vi "ClassAttributes_AddClassAttributes.vi"(7 "Action":T3=enum."GeneratePattern", 8 "error in (no error)":errorcluster, 10 "DataIn":variant, 11 "ClassRefToActOn":refnum<vi>) -> (0 "error out":errorcluster, 1 "Name":string, 2 "DataOut":variant, 3 "Cancelled":bool)   [LabVIEW 2012]
uses:
  <resource>/Framework/Providers/Open_GDS/ClassProviders/Provider_BaseClassInterface/BaseProvider_SubVIs/BaseProvider_DesignPatternsActions.ctl
  <resource>/Framework/Providers/Open_GDS/ClassProviders/Common/CommonVIs/CommonVIs_AttributeDataType.ctl
  <resource>/Framework/Providers/Open_GDS/ClassProviders/Common/LvClass_class/GDSLvClass_ProviderTypes.ctl
  <resource>/Framework/Providers/Open_GDS/ClassProviders/Common/ScriptingFunctions/Scripting_ConnectorPanePatternType.ctl
  <vilib>/picture/picture.llb/imagedata.ctl
  <resource>/Framework/Providers/Open_GDS/ClassProviders/Provider_LvNativeClass/ClassWriterNative_class/ClassWriterNative.lvclass
  <resource>/Framework/Providers/Open_GDS/ClassProviders/Provider_BaseClassInterface/CreateMethodData.ctl
  <resource>/Framework/Providers/Open_GDS/ClassProviders/Provider_EndevoGOOP300/GOOP300_SubVIs/GOOP300_MethodScopeType.ctl
  <resource>/Framework/Providers/Open_GDS/ClassProviders/Provider_LvNativeClass/ClassWriterNative_class/IconDetails.ctl
  <resource>/Framework/Providers/Open_GDS/ClassProviders/Provider_LvNativeClass/ClassWriterNative_class/IconSize.ctl
  <resource>/Framework/Providers/Open_GDS/ClassProviders/Provider_BaseClassInterface/ClassWriter_class/ClassWriter.lvclass
panel:
  in  "_Cancel":bool
  in  "_OK":bool
  in  "ProcessName":T2(array[cluster]) caption="Attributes to add (can be empty)\nName                                              Array?      Data Type" {"Array?" items=["No", "1D", "2D", "3D"]}
  # "Class Attributes"
  # "Create"
  # "Get"
  # "Set"
  # "method"
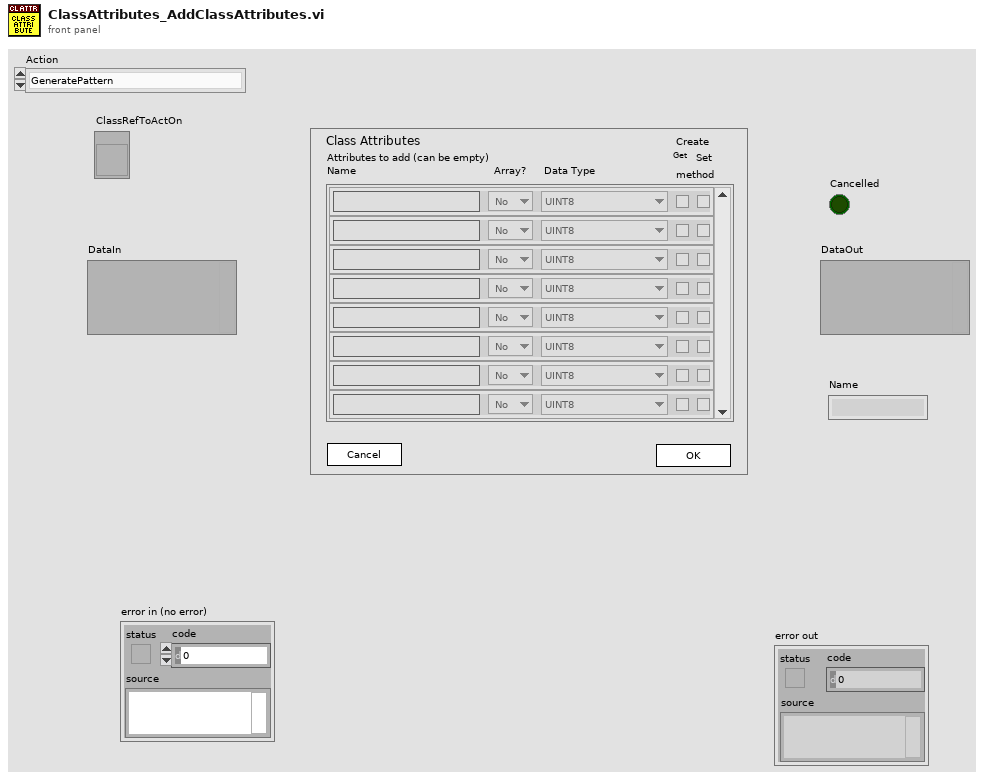
[diagram p1: front panel]
types:
  T1 = typedef "CommonVIs_AttributeDataType.ctl" = enum16{"UINT8", "INT8", "UINT16", "INT16", "UINT32", "INT32", "UINT64", "INT64", "SGL", "DBL", "EXT", "CSG", "CDB", "CXT", "TimeStamp", "STRING", "PATH", "BOOL", "ENUM", "RefNum", "VIRefNum", "ClassRefNum", "Cluster", "Variant", "TypeRef", "Waveform", "LabVIEW Object", "Other"}
  T2 = cluster{"Name":string, "Array?":u16, "AttributeDataType":T1, "GetMethod":bool, "SetMethod":bool}[]
  T3 = typedef "BaseProvider_DesignPatternsActions.ctl" = enum16{"AddPatternDialog", "GeneratePattern", "RemovePattern", "CreatePatternMethod", "UpdatePattern"}
  T4 = typedef "GDSLvClass_ProviderTypes.ctl" = enum16{"UnKnown(LabVOOP)", "Native", "EndevoGOOP3", "OpenG(RootObject)", "OpenG(OpenG_Object)", "EndevoGOOP4", "JKI1"}
  T5 = cluster{"Application":refnum<vi>, "SupportFolder":path, "TemplateName":string, "ClassProvider":T4, "ProtectedFolder":path, "UtilsFolder":path, "ProtectedFolderRef":refnum<vi>, "UtilsFolderRef":refnum<vi>, "ClassName":string, "GetClassAttributes.vi":path, "ClassAttributes.ctl":path, "GetClassAttributesRef":refnum<vi>, "ClassAttributesRef":refnum<vi>, "ProcessIdRef":refnum<vi>, "Data":cluster{"Name":string, "Array?":u16, "AttributeDataType":T1, "GetMethod":bool, "SetMethod":bool}[], "Singleton":bool, "VI_ToFind":path, "MethodTemplate":path, "VI":refnum<vi>, "GetObjectStatus":path}
  T6 = cluster{"ProcessName":cluster{"Name":string, "Array?":u16, "AttributeDataType":T1, "GetMethod":bool, "SetMethod":bool}[]}
  T7 = cluster{"Cancelled":bool, "Files":path[], "ClassPath":path, "DataOut":variant}
  T8 = enum32{"invalid lock state", "Not Locked", "Locked (No Password)", "Password-protected"}
  T9 = typedef "imagedata.ctl" = cluster{"image type":i32, "image depth":i32, "image":u8[], "mask":u8[], "colors":u32[], "Rectangle":cluster{"left":i16, "top":i16, "right":i16, "bottom":i16}}
  T10 = typedef "ClassWriter.lvclass/CreateMethodData.ctl" = cluster{"MethodName":string, "RelativeMethodPath":path, "MethodDescription":string, "Scope/Visibility":T11, "MethodTemplateName":string, "IconOut":u8[][], "RelativeProjectClassPath":string, "OpenViAfterCreation":bool, "DynamicDispatchVi":bool, "ExtraCreateParameters":variant, "MustOverride":bool, "MustCallParent":bool, "IconDetails":T12, "AF-Option":variant, "TemplatePath":path}
  T11 = typedef "GOOP300_MethodScopeType.ctl" = enum16{"Use Parent Folder Scope", "Public", "Protected", "Private", "Community"}
  T12 = typedef "ClassWriterNative.lvclass/IconDetails.ctl" = cluster{"IconSize":T13, "ImageRows(32)":i32, "ConnectorPaneHeight":i32[]}
  T13 = typedef "ClassWriterNative.lvclass/IconSize.ctl" = enum16{"Full", "1 c-term high", "2 c-term high", "3 c-term high"}
  T14 = typedef "GDSLvCLass_ClassSettingsType.ctl" = cluster{"ClassProviderName":string, "ClassTemplateUsed":string, "ClassTemplateVersion":string, "ClassDescription":string, "PlugIns":T15[], "ConnectorPanePattern":string}
  T15 = typedef "GDSLvClass_PlugIn.ctl" = cluster{"Type":T16, "ID":string, "Version":string, "Path":path, "Name":string, "Data":variant}
  T16 = typedef "GDSLvClass_PlugInTypes.ctl" = enum16{"DesignPattern", "MethodTypes"}
  T17 = enum32{"invalid scope", "public", "private", "protected"}[]
  T18 = typedef "Scripting_ConnectorPanePatternType.ctl" = u16
  T19 = typedef "GDSLvClass_IconSettingsType.ctl" = cluster{"Frame":u32, "Frame thickness":u8, "Header Background":u32, "Header Text":u32, "ColorPublic":u32, "ColorProtected":u32, "ColorPrivate":u32, "Body Text":u32, "ClassBodyIcon":string}
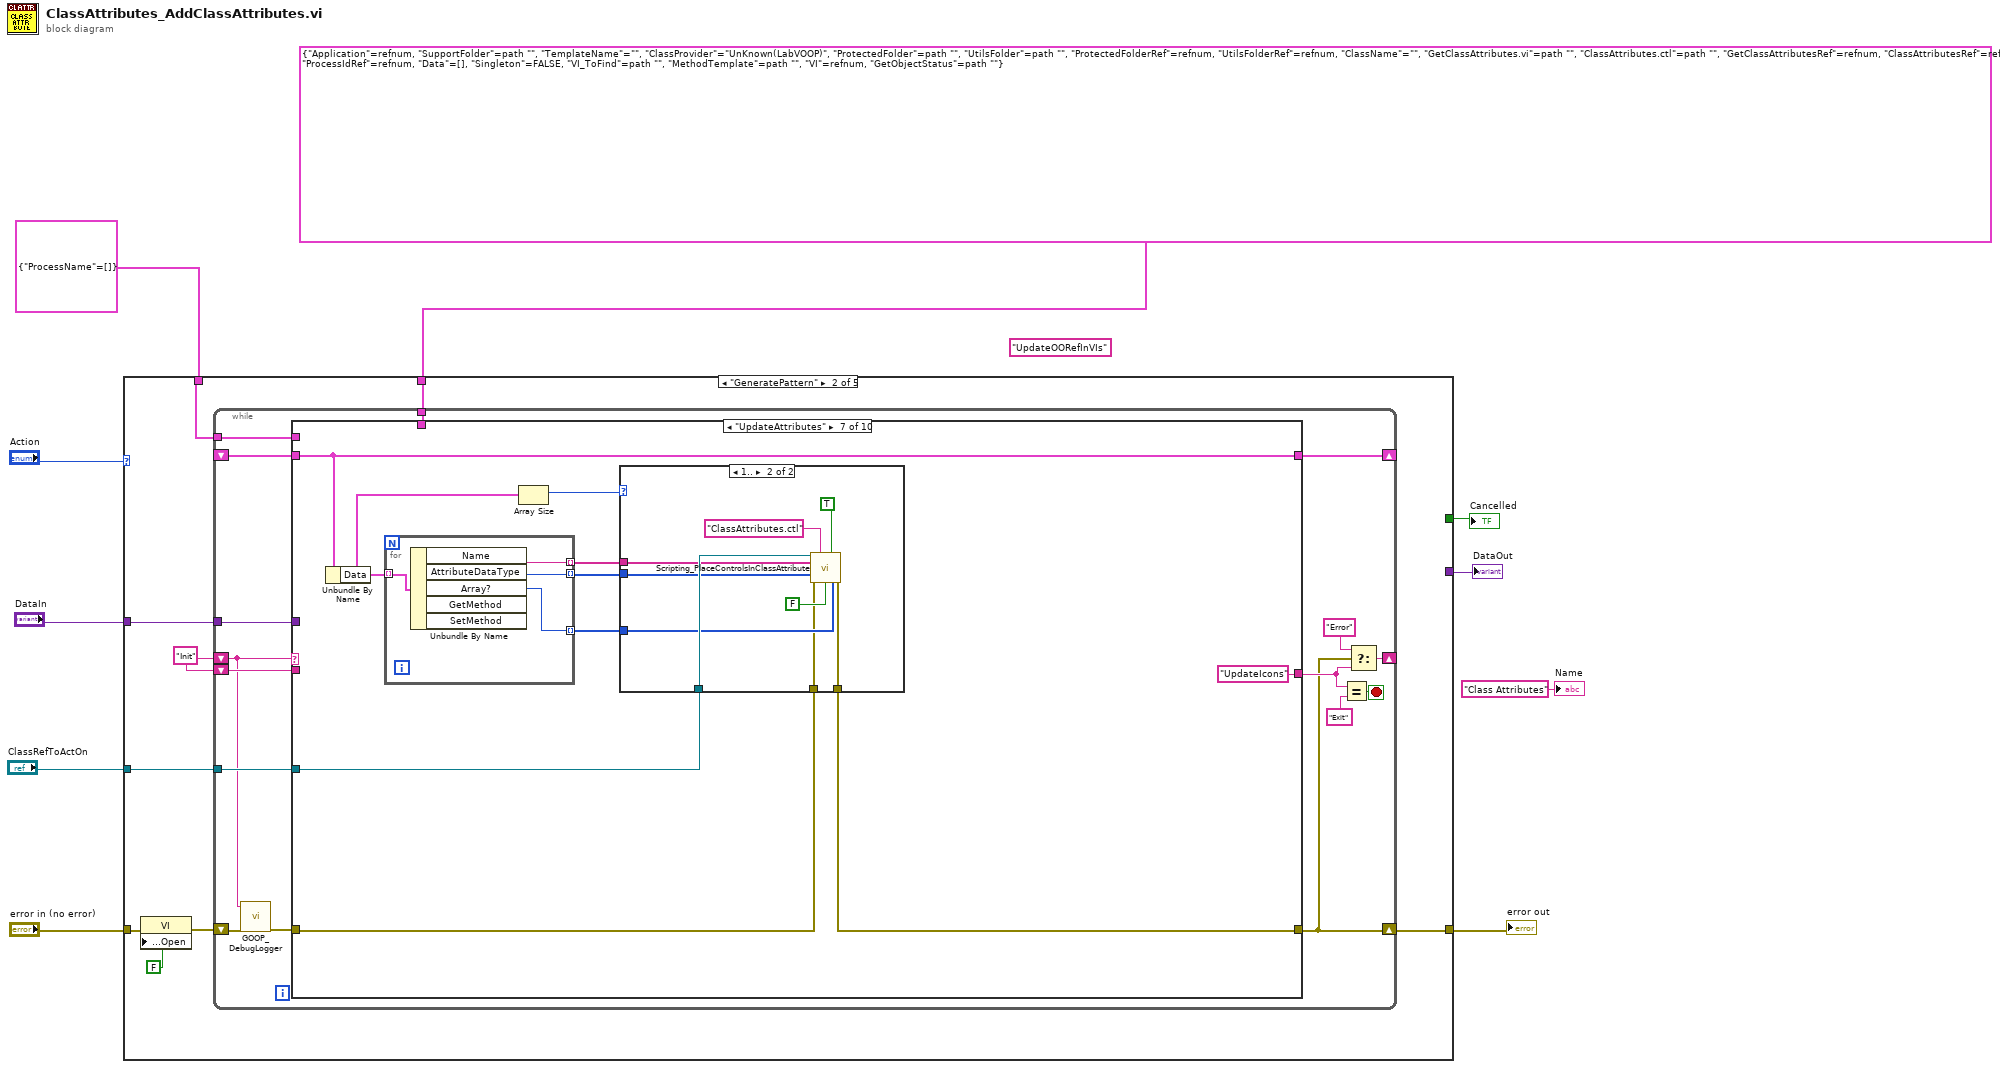
[diagram p0: block diagram]
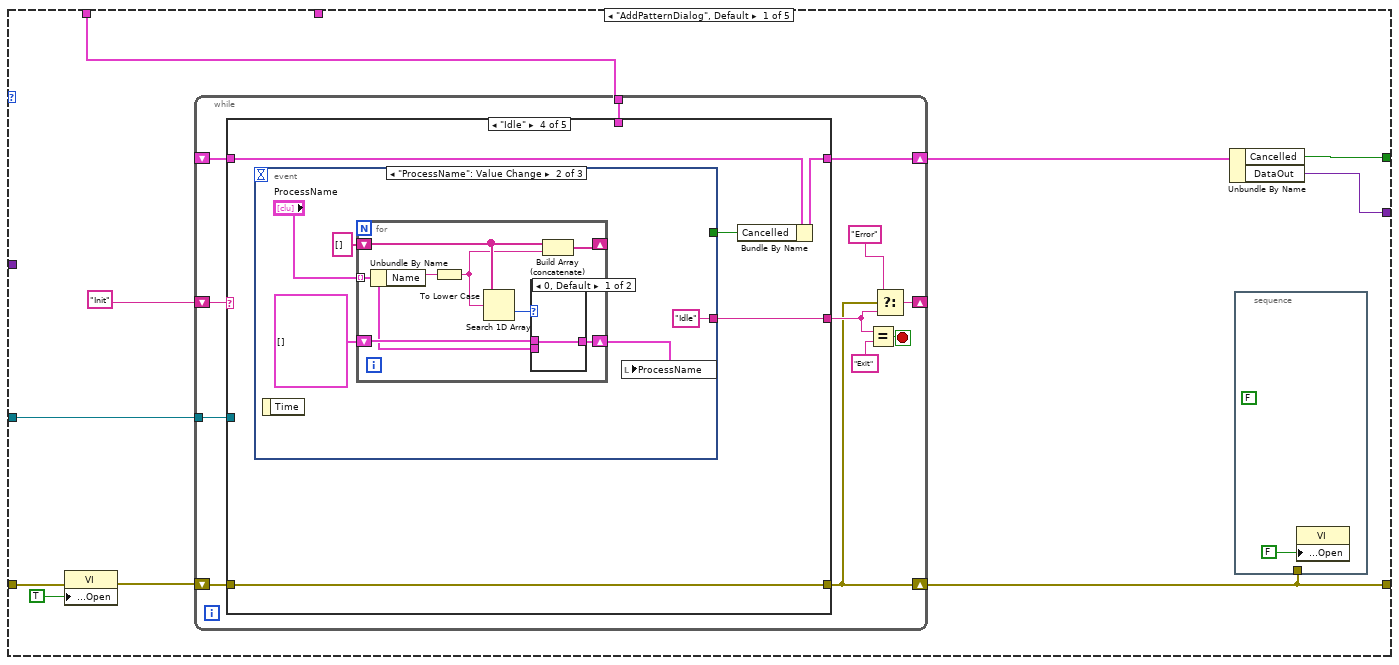
[diagram p2: hidden frame]
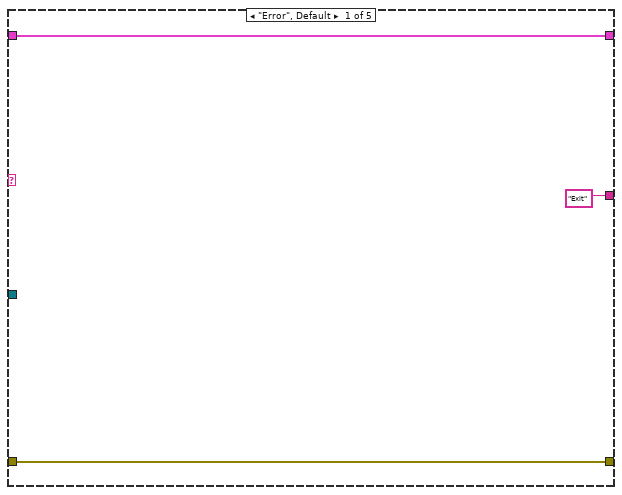
[diagram p3: hidden frame]
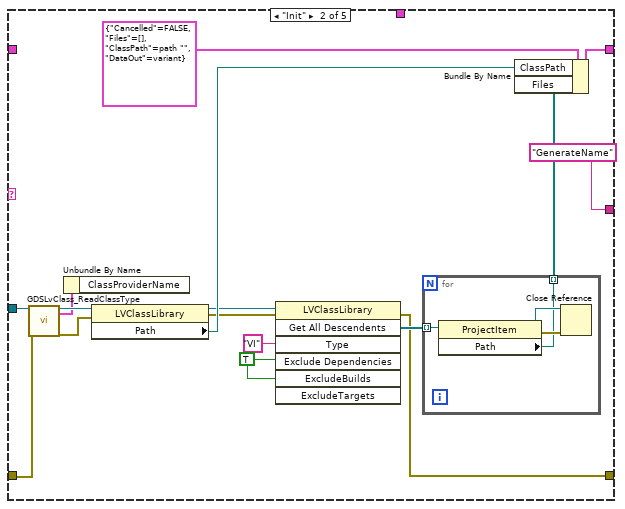
[diagram p4: hidden frame]
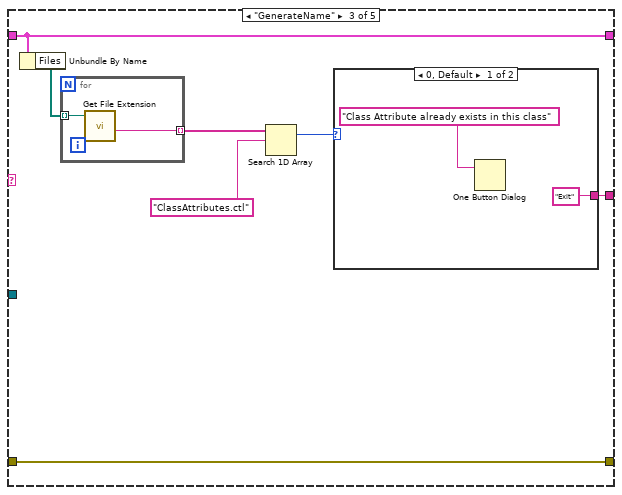
[diagram p5: hidden frame]
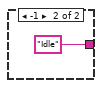
[diagram p6: hidden frame]
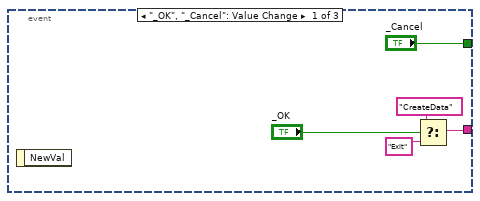
[diagram p7: hidden frame]
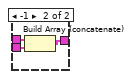
[diagram p8: hidden frame]
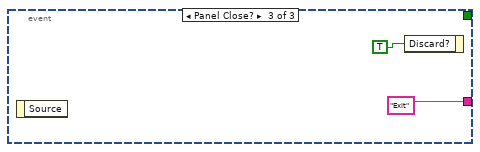
[diagram p9: hidden frame]
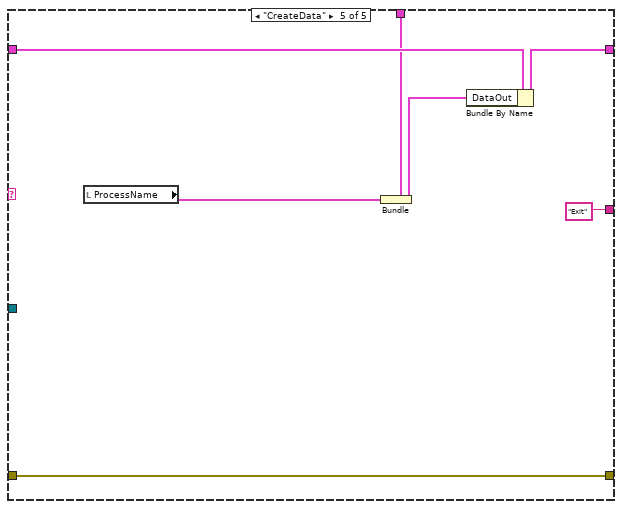
[diagram p10: hidden frame]
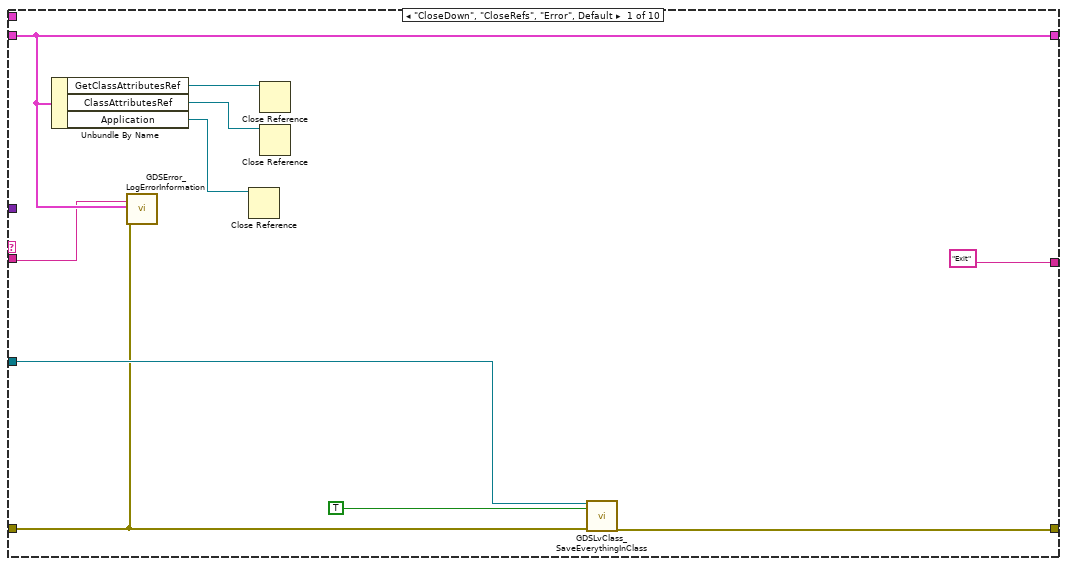
[diagram p11: hidden frame]
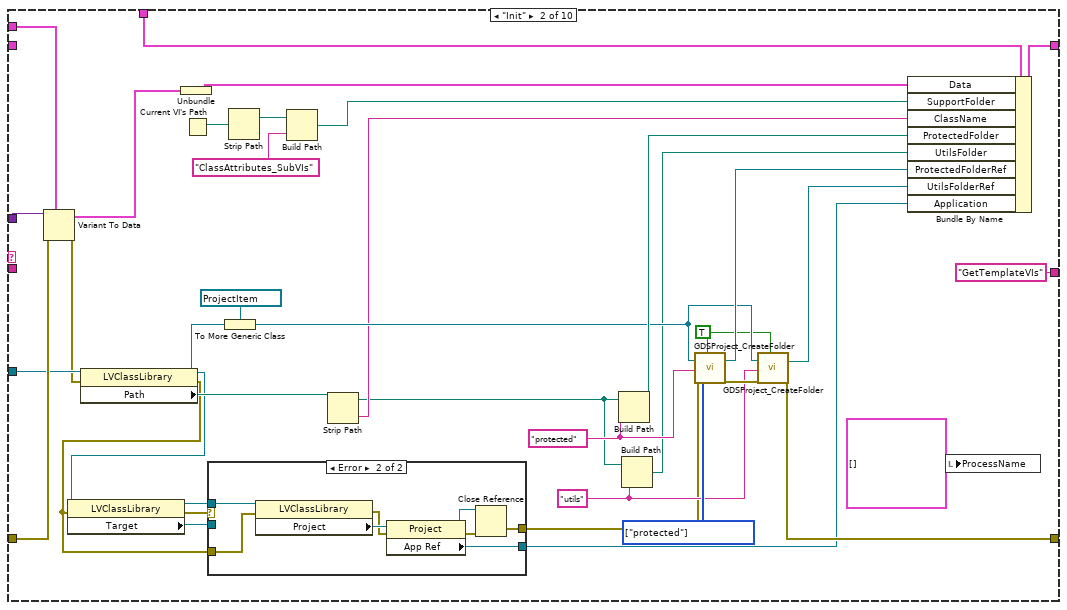
[diagram p12: hidden frame]
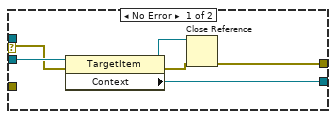
[diagram p13: hidden frame]
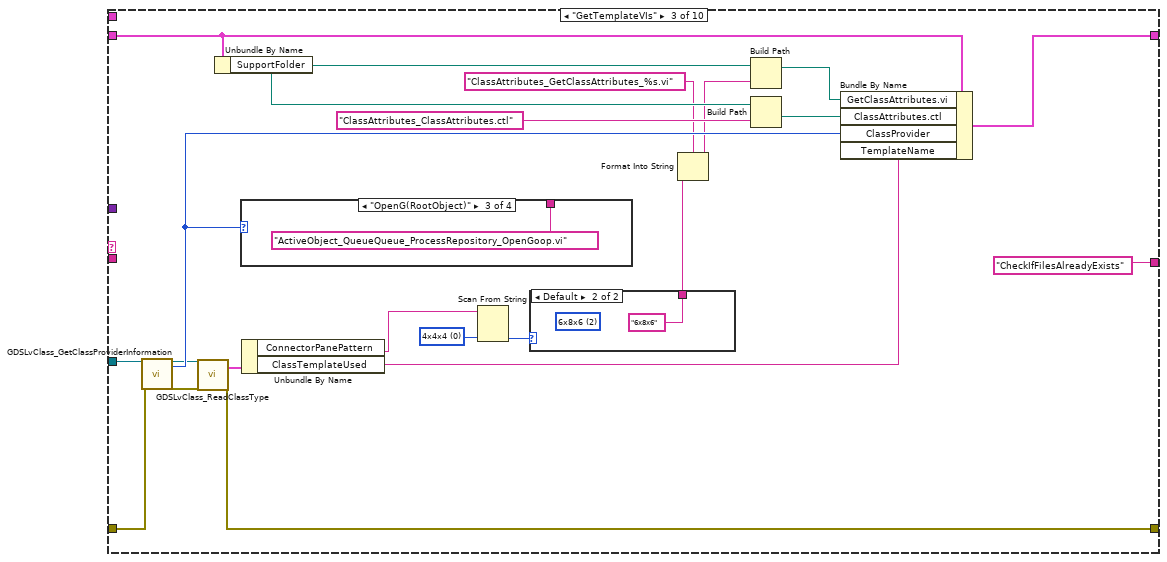
[diagram p14: hidden frame]
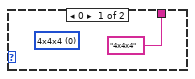
[diagram p15: hidden frame]
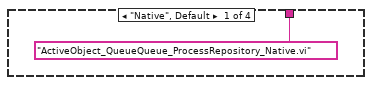
[diagram p16: hidden frame]
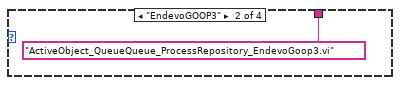
[diagram p17: hidden frame]
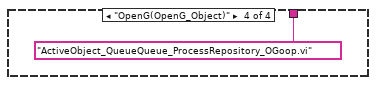
[diagram p18: hidden frame]
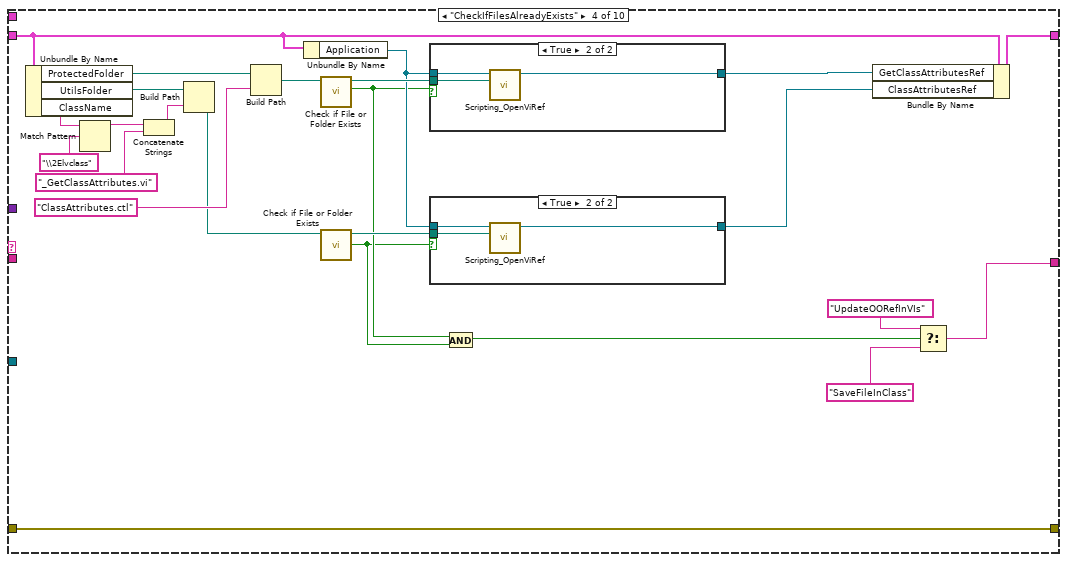
[diagram p19: hidden frame]
diagram:
  (unwired) "UpdateOORefInVIs"
  n1 = case shown="\"GeneratePattern\"" "Action" {
    tunnel: "error in (no error)" -> [w19 w107 w531 w622 w623]
    tunnel: [w16 w113 w537 w622 w623] -> w8
    tunnel: "ClassRefToActOn" -> [w14 w109 w533 _ _]
    tunnel: [w13 _ _ _ _] -> w6
    tunnel: [w12 _ _ _ _] -> w5
    tunnel: T6 {"ProcessName"=[]} ("output cluster") -> [w11 w111 w535 _ _]
    tunnel: "DataIn" -> [_ w112 w536 _ _]
    tunnel: T5 {"Application"=refnum, "SupportFolder"=path "", "TemplateName"="", "ClassProvider"=enum."UnKnown(LabVOOP)", "ProtectedFolder"=path "", "UtilsFolder"=path "", "ProtectedFolderRef"=refnum, "UtilsFolderRef"=refnum, "ClassName"="", "GetClassAttributes.vi"=path "", "ClassAttributes.ctl"=path "", "GetClassAttributesRef"=refnum, "ClassAttributesRef"=refnum, "ProcessIdRef"=refnum, "Data"=[], "Singleton"=FALSE, "VI_ToFind"=path "", "MethodTemplate"=path "", "VI"=refnum, "GetObjectStatus"=path ""} -> [_ w110 w534 _ _]
    frame "AddPatternDialog", Default {
      n2 = property class="VI"(error in=w19, "Front Panel.Open"=TRUE ("Front Panel Window:Open")) -> (error out=w18:errorcluster)  [unwired: 1 in, 1 out]
      n3 = while {
        shift-right: [w26] -> w16
        shift-left: w18 -> [w33]
        shift-right: [w31] -> _
        shift-left: "Init" -> [w32]
        shift-right: [w25] -> w15
        shift-left: _ -> [w24]
        tunnel: w14 -> [w23]
        tunnel: w11 -> [w22]
        stop <- w30 stop-if-true
        n4 = case shown="\"Idle\"" w32 {
          tunnel: w33 -> [w36 w39 w60 w72 w100]
          tunnel: [w36 w48 w60 w72 w100] -> w26
          tunnel: ["Exit" "GenerateName" w62 w73 "Exit"] -> w27
          tunnel: [w34 w46 w61 w71 w102] -> w25
          tunnel: w24 -> [w34 _ w61 w69 w104]
          tunnel: w23 -> [_ w41 _ _ _]
          tunnel: w22 -> [_ _ _ _ w99]
          frame "Error", Default {
          }
          frame "Init" {
            w50 = TRUE ("ExcludeDependencies")
            n5 = call <resource>:"GDSLvClass_ReadClassType.vi"("Class Refnum In"=w41, "error in (no error)"=w39) -> ("Class Refnum Out"=w40:refnum<vi>, "ClassSettings"=w37:T14, "error out"=w38:errorcluster)  [unwired: 15 in]
            n6 = Unbundle By Name(w37) -> ()  [unwired: 1 out]
            n7 = property class="LVClassLibrary"(reference=w40, error in=w38) -> (reference out=w43:refnum<vi>, error out=w42:errorcluster, "Path"=w45:path)
            n8 = invoke class="LVClassLibrary" method="Get All Descendents"(reference=w43, error in=w42, "Type"="VI", "Exclude Dependencies"=w50, "ExcludeBuilds"=w50) -> (error out=w48:errorcluster, "All Descendents"=w49:refnum<vi>[])  [unwired: 2 in, 5 out]
            n9 = for {
              tunnel: w49 -> [w56] mode=indexing
              tunnel: [w53] -> w44 mode=indexing
              n10 = property class="ProjectItem"(reference=w56) -> (reference out=w54:refnum<vi>, error out=w55:errorcluster, "Path"=w53:path)  [unwired: 1 in]
              n11 = Close Reference(reference=w54, error in (no error)=w55) -> ()  [unwired: 1 out]
            }
            n12 = Bundle By Name(cluster=T7 {"Cancelled"=FALSE, "Files"=[], "ClassPath"=path "", "DataOut"=variant}, "ClassPath"=w45, "Files"=w44) -> (w46:T7)
          }
          frame "GenerateName" {
            n13 = Unbundle By Name(w61) -> ("Files"=w63:path[])
            n14 = for {
              tunnel: w63 -> [w68] mode=indexing
              tunnel: [w67] -> w59 mode=indexing
              n15 = call <vilib>:"Get File Extension.vi"("file"=w68) -> ("filename without extension"=w67:string)  [unwired: 7 in, 3 out]
            }
            n16 = Search 1D Array(1D array=w59, element="ClassAttributes.ctl") -> (index of element=w57:i32)  [unwired: 1 in]
            n17 = case shown="0, Default" w57 {
              tunnel: ["Exit" "Idle"] -> w62
              frame 0, Default {
                n18 = One Button Dialog(message="Class Attribute already exists in this class") -> ()  [unwired: 1 in, 1 out]
              }
              frame -1 {
              }
            }
          }
          frame "Idle" {
            n19 = event shown="[1] \"ProcessName\": Value Change" {
              selector: _ -> [_ _ _]
              dyn-events: _ -> [_ _ _]
              timeout: _ -> [_ _ _]
              tunnel: [w77 "Idle" "Exit"] -> w73
              tunnel: ["_Cancel" _ _] -> w70
              event "_OK", "_Cancel": Value Change {
                n20 = event-data() -> ()  [unwired: 1 in, 1 out]
                n21 = Select(t="CreateData", s="_OK", f="Exit") -> (s? t:f=w77:string)
              }
              event "ProcessName": Value Change {
                n22 = event-data() -> ()  [unwired: 1 in, 1 out]
                n23 = for {
                  tunnel: "ProcessName" -> [w85] mode=indexing
                  shift-right: [w91] -> _
                  shift-left: string[] [] -> [w89]
                  shift-right: [w84] -> w79
                  shift-left: T2 [] -> [w86]
                  n24 = Unbundle By Name(w85) -> ("Name"=w90:string)
                  n25 = To Lower Case(string=w90) -> (all lower case string=w88:string)
                  n26 = Search 1D Array(1D array=w89, element=w88) -> (index of element=w87:i32)  [unwired: 1 in]
                  n27 = case shown="0, Default" w87 {
                    tunnel: w86 -> [w92 w95]
                    tunnel: w85 -> [_ w94]
                    tunnel: [w92 w93] -> w84
                    frame 0, Default {
                    }
                    frame -1 {
                      n28 = Build Array (concatenate)(w95, w94) -> (w93:T2)
                    }
                  }
                  n29 = Build Array (concatenate)(w89, w88) -> (w91:string[])
                }
                n30 = local write "ProcessName"(w79) -> ()
              }
              event Panel Close? {
                n31 = event-data() -> ()  [unwired: 1 in, 1 out]
                n32 = event-data("Discard?"=TRUE) -> ()  [unwired: 1 in, 1 out]
              }
            }
            n33 = Bundle By Name(cluster=w69, "Cancelled"=w70) -> (w71:T7)
          }
          frame "CreateData" {
            n34 = local read "ProcessName"() -> (w98:T2)
            n35 = Bundle(cluster=w99, "ProcessName"=w98) -> (w103:T6)
            n36 = Bundle By Name(cluster=w104, "DataOut"=w103) -> (w102:T7)
          }
        }
        n37 = Equal?(x=w27, y="Exit") -> (x = y?=w30:bool)
        n38 = Select(t="Error", s=w26, f=w27) -> (s? t:f=w31:string)
      }
      n39 = Unbundle By Name(w15) -> ("Cancelled"=w13:bool, "DataOut"=w12:variant)
      n40 = stacked-sequence {
        tunnel: w16 -> [_]
        frame #0 {
          (unwired) FALSE ("Visible")
          n41 = property class="VI"("Front Panel.Open"=FALSE ("Front Panel Window:Open")) -> ()  [unwired: 2 in, 2 out]
        }
      }
    }
    frame "GeneratePattern" {
      w105 = "Init"
      n42 = property class="VI"(error in=w107, "Front Panel.Open"=FALSE ("Front Panel Window:Open")) -> (error out=w106:errorcluster)  [unwired: 1 in, 1 out]
      n43 = while {
        shift-right: [w124] -> w113
        shift-left: w106 -> [w116]
        shift-right: [w129] -> _
        shift-left: w105 -> [w114]
        shift-right: [w123] -> _
        shift-left: _ -> [w122]
        tunnel: w112 -> [w121]
        tunnel: w111 -> [w120]
        tunnel: w110 -> [w119]
        tunnel: w109 -> [w118]
        shift-left: w105 -> [w117]
        stop <- w128 stop-if-true
        n44 = call <resource>:"GOOP_DebugLogger.vi"("error in (no error)"=w116, "State"=w114) -> ("error out"=w115:errorcluster)  [unwired: 9 in]
        n45 = case shown="\"UpdateAttributes\"" w114 {
          tunnel: w115 -> [w130 w171 w209 w232 w274 w303 w312 w336 w389 w476]
          tunnel: [w135 w156 w202 w232 w276 w297 w311 w335 w386 w461] -> w124
          tunnel: ["Exit" "GetTemplateVIs" "CheckIfFilesAlreadyExists" w218 "UpdateOORefInVIs" "UpdateAttributes" "UpdateIcons" "CreateMethods" w381 "CloseRefs"] -> w125
          tunnel: [w132 w175 w205 w228 w291 w304 w317 w338 w378 w460] -> w123
          tunnel: w122 -> [w132 _ w208 w229 w259 w304 w317 w338 w379 w460]
          tunnel: w121 -> [_ w174 _ _ _ _ _ _ _ _]
          tunnel: w120 -> [_ w173 _ _ _ _ _ _ _ _]
          tunnel: w119 -> [_ w172 _ _ _ _ _ _ _ _]
          tunnel: w118 -> [w134 w170 w210 _ _ w302 w316 w340 w385 w475]
          tunnel: w117 -> [w131 _ _ _ _ _ _ _ _ _]
          frame "CloseDown", "CloseRefs", "Error", Default {
            n46 = Unbundle By Name(w132) -> ("GetClassAttributesRef"=w138:refnum<vi>, "ClassAttributesRef"=w137:refnum<vi>, "Application"=w133:refnum<vi>)
            n47 = call <resource>:"GDSError_LogErrorInformation.vi"("State"=w131, "LocalVariableData"=w132, "error in (no error)"=w130) -> ()  [unwired: 16 in, 1 out]
            n48 = Close Reference(reference=w133) -> ()  [unwired: 1 in, 1 out]
            n49 = Close Reference(reference=w138) -> ()  [unwired: 1 in, 1 out]
            n50 = Close Reference(reference=w137) -> ()  [unwired: 1 in, 1 out]
            n51 = call <resource>:"GDSLvClass_SaveEverythingInClass.vi"("ClassRefIn"=w134, "ForceResaving(False)"=TRUE, "error in"=w130) -> ("error out"=w135:errorcluster)  [unwired: 15 in, 1 out]
          }
          frame "Init" {
            w151 = "utils" ("name or relative path")
            w168 = T17 [enum."protected"] items=["invalid scope", "public", "private", "protected"] ("FolderScope")
            w157 = TRUE ("CreateThePhysicalFolderIfPossible(False)")
            w167 = "protected" ("name or relative path")
            n52 = Variant To Data(error in=w171, type=w173, Variant=w174) -> (data=w150:T6, error out=w162:errorcluster)
            n53 = property class="LVClassLibrary"(reference=w170, error in=w162) -> (reference out=w143:refnum<vi>, error out=w140:errorcluster, "Path"=w160:path)
            n54 = property class="LVClassLibrary"(reference=w143, error in=w140) -> (reference out=w146:refnum<vi>, error out=w144:errorcluster, "Target"=w145:refnum<vi>)
            n55 = Unbundle(w150) -> ("ProcessName"=w149:T2)
            n56 = Current VI's Path() -> (path=w165:path)
            n57 = case shown="Error" w144 {
              selector: w144 -> [w178 _]
              tunnel: w145 -> [w182 _]
              tunnel: [w181 w184] -> w142
              tunnel: [w177 w185] -> w141
              tunnel: w146 -> [_ w190]
              tunnel: w140 -> [_ w189]
              frame No Error {
                n58 = property class="TargetItem"(reference=w182, error in=w178) -> (reference out=w179:refnum<vi>, error out=w180:errorcluster, "Context"=w181:refnum<vi>)
                n59 = Close Reference(reference=w179, error in (no error)=w180) -> (error out=w177:errorcluster)
              }
              frame Error {
                n60 = property class="LVClassLibrary"(reference=w190, error in=w189) -> (error out=w183:errorcluster, "Project"=w188:refnum<vi>)  [unwired: 1 out]
                n61 = property class="Project"(reference=w188, error in=w183) -> (reference out=w186:refnum<vi>, error out=w187:errorcluster, "App Ref"=w184:refnum<vi>)
                n62 = Close Reference(reference=w186, error in (no error)=w187) -> (error out=w185:errorcluster)
              }
            }
            n63 = To More Generic Class(target class=refnum<vi> refnum ("AddItem"), reference=w143) -> (generic class reference=w158:refnum<vi>)
            n64 = Strip Path(path=w165) -> (stripped path=w164:path)  [unwired: 1 out]
            n65 = Build Path(base path=w164, name or relative path="ClassAttributes_SubVIs") -> (appended path=w155:path)
            n66 = Strip Path(path=w160) -> (stripped path=w147:path, name=w152:string)
            n67 = Build Path(base path=w147, name or relative path=w167) -> (appended path=w166:path)
            n68 = Build Path(base path=w147, name or relative path=w151) -> (appended path=w153:path)
            n69 = call <resource>:"GDSProject_CreateFolder.vi"("Project Item To Create Folder Below(Use MyComputer if not wired)"=w158, "FolderName"=w167, "error in (no error)"=w141, "FolderScope"=w168, "CreateThePhysicalFolderIfPossible(False)"=w157) -> ("ItemOut"=w161:refnum<vi>, "error out"=w159:errorcluster)  [unwired: 11 in, 2 out]
            n70 = call <resource>:"GDSProject_CreateFolder.vi"("Project Item To Create Folder Below(Use MyComputer if not wired)"=w158, "FolderName"=w151, "error in (no error)"=w159, "CreateThePhysicalFolderIfPossible(False)"=w157) -> ("ItemOut"=w154:refnum<vi>, "error out"=w156:errorcluster)  [unwired: 12 in, 2 out]
            n71 = Bundle By Name(cluster=w172, "Data"=w149, "SupportFolder"=w155, "ClassName"=w152, "ProtectedFolder"=w166, "UtilsFolder"=w153, "ProtectedFolderRef"=w161, "UtilsFolderRef"=w154, "Application"=w142) -> (w175:T5)
            n72 = local write "ProcessName"(T2 [] ("ProcessName")) -> ()
          }
          frame "GetTemplateVIs" {
            w196 = T18 0 items=["4x4x4", "5x6x5", "6x8x6"] ("Pattern")
            n73 = call <resource>:"GDSLvClass_GetClassProviderInformation.vi"("Class Refnum In"=w210, "error in (no error)"=w209) -> ("Class Refnum Out"=w204:refnum<vi>, "ClassProvider"=w206:T4, "error out"=w203:errorcluster)  [unwired: 15 in]
            n74 = call <resource>:"GDSLvClass_ReadClassType.vi"("Class Refnum In"=w204, "error in (no error)"=w203) -> ("ClassSettings"=w201:T14, "error out"=w202:errorcluster)  [unwired: 15 in, 1 out]
            n75 = Unbundle By Name(w208) -> ("SupportFolder"=w199:path)
            n76 = case shown="\"OpenG(RootObject)\"" w206 {
              tunnel: ["ActiveObject_QueueQueue_ProcessRepository_Native.vi" ("name or relative path") "ActiveObject_QueueQueue_ProcessRepository_EndevoGoop3.vi" ("name or relative path") "ActiveObject_QueueQueue_ProcessRepository_OpenGoop.vi" ("name or relative path") "ActiveObject_QueueQueue_ProcessRepository_OGoop.vi" ("name or relative path")] -> _
              frame "Native", Default {
              }
              frame "EndevoGOOP3" {
              }
              frame "OpenG(RootObject)" {
              }
              frame "OpenG(OpenG_Object)" {
              }
            }
            n77 = Unbundle By Name(w201) -> ("ConnectorPanePattern"=w192:string, "ClassTemplateUsed"=w200:string)
            n78 = Scan From String(input string=w192, default 1=w196) -> (output 1=w193:T18)  [unwired: 3 in, 3 out]
            n79 = case shown="Default" w193 {
              tunnel: ["4x4x4" "6x8x6"] -> w191
              frame 0 {
                (unwired) T18 0 items=["4x4x4", "5x6x5", "6x8x6"] ("Pattern")
              }
              frame Default {
                (unwired) T18 2 items=["4x4x4", "5x6x5", "6x8x6"] ("Pattern")
              }
            }
            n80 = Format Into String(format string="ClassAttributes_GetClassAttributes_%s.vi" ("name or relative path"), w191) -> (resulting string=w194:string)  [unwired: 2 in, 1 out]
            n81 = Build Path(base path=w199, name or relative path=w194) -> (appended path=w207:path)
            n82 = Build Path(base path=w199, name or relative path="ClassAttributes_ClassAttributes.ctl") -> (appended path=w197:path)
            n83 = Bundle By Name(cluster=w208, "GetClassAttributes.vi"=w207, "ClassAttributes.ctl"=w197, "ClassProvider"=w206, "TemplateName"=w200) -> (w205:T5)
          }
          frame "CheckIfFilesAlreadyExists" {
            n84 = Unbundle By Name(w229) -> ("ProtectedFolder"=w235:path, "UtilsFolder"=w241:path, "ClassName"=w240:string)
            n85 = Match Pattern(string=w240, regular expression="\\2Elvclass") -> (before substring=w238:string)  [unwired: 1 in, 3 out]
            n86 = Concatenate Strings(w238, "_GetClassAttributes.vi" ("string")) -> (w236:string)
            n87 = Build Path(base path=w241, name or relative path=w236) -> (appended path=w231:path)
            n88 = Build Path(base path=w235, name or relative path="ClassAttributes.ctl") -> (appended path=w233:path)
            n89 = Unbundle By Name(w229) -> ("Application"=w225:refnum<vi>)
            n90 = call <vilib>:"Check if File or Folder Exists.vi"("path"=w233) -> ("file or folder exists?"=w223:bool, "dup path"=w230:path)  [unwired: 8 in, 1 out]
            n91 = call <vilib>:"Check if File or Folder Exists.vi"("path"=w231) -> ("file or folder exists?"=w222:bool, "dup path"=w226:path)  [unwired: 8 in, 1 out]
            n92 = case shown="True" w223 {
              tunnel: w225 -> [_ w247]
              tunnel: w230 -> [_ w246]
              tunnel: [_ w245] -> w227
              frame False {
              }
              frame True {
                n93 = call <resource>:"Scripting_OpenViRef.vi"("ViPath/ViName"=w246, "AppRef"=w247) -> ("vi reference"=w245:refnum<vi>)  [unwired: 8 in, 1 out]
              }
            }
            n94 = case shown="True" w222 {
              tunnel: w225 -> [_ w244]
              tunnel: w226 -> [_ w243]
              tunnel: [_ w242] -> w224
              frame False {
              }
              frame True {
                n95 = call <resource>:"Scripting_OpenViRef.vi"("ViPath/ViName"=w243, "AppRef"=w244) -> ("vi reference"=w242:refnum<vi>)  [unwired: 8 in, 1 out]
              }
            }
            n96 = And(x=w223, y=w222) -> (x .and. y?=w221:bool)
            n97 = Bundle By Name(cluster=w229, "GetClassAttributesRef"=w227, "ClassAttributesRef"=w224) -> (w228:T5)
            n98 = Select(t="UpdateOORefInVIs", s=w221, f="SaveFileInClass") -> (s? t:f=w218:string)
          }
          frame "SaveFileInClass" {
            w260 = 1357 ("code")
            n99 = Unbundle By Name(w259) -> ("Application"=w268:refnum<vi>)
            n100 = Unbundle By Name(w259) -> ("ProtectedFolderRef"=w278:refnum<vi>, "UtilsFolderRef"=w289:refnum<vi>, "ProtectedFolder"=w280:path, "UtilsFolder"=w292:path, "ClassName"=w287:string)
            n101 = Unbundle By Name(w259) -> ("GetClassAttributes.vi"=w273:path, "ClassAttributes.ctl"=w269:path)
            n102 = Match Pattern(string=w287, regular expression="\\2Elvclass") -> (before substring=w285:string)  [unwired: 1 in, 3 out]
            n103 = call <resource>:"Scripting_OpenViRef.vi"("error in"=w274, "ViPath/ViName"=w273, "AppRef"=w268) -> ("error out"=w272:errorcluster, "vi reference"=w267:refnum<vi>)  [unwired: 7 in]
            n104 = Concatenate Strings(w285, "_GetClassAttributes.vi" ("string")) -> (w283:string)
            n105 = call <resource>:"Scripting_OpenViRef.vi"("error in"=w272, "ViPath/ViName"=w269, "AppRef"=w268) -> ("error out"=w271:errorcluster, "vi reference"=w270:refnum<vi>)  [unwired: 7 in]
            n106 = Build Path(base path=w292, name or relative path=w283) -> (appended path=w281:path)
            n107 = invoke class="VI" method="Save.Instrument"(reference=w267, error in=w271, "Path to saved file"=w281) -> (reference out=w282:refnum<vi>, error out=w265:errorcluster)  [unwired: 3 in, 4 out]
            n108 = Build Path(base path=w280, name or relative path="ClassAttributes.ctl") -> (appended path=w266:path)
            n109 = call <resource>:"Error_ClearError.vi"("code"=w260, "error in (no error)"=w265) -> ("error out"=w264:errorcluster)  [unwired: 16 in, 1 out]
            n110 = invoke class="VI" method="Save.Instrument"(reference=w270, error in=w264, "Path to saved file"=w266) -> (error out=w263:errorcluster)  [unwired: 3 in, 5 out]
            n111 = call <resource>:"Error_ClearError.vi"("code"=w260, "error in (no error)"=w263) -> ("error out"=w262:errorcluster)  [unwired: 16 in, 1 out]
            n112 = invoke class="ProjectItem" method="AddFile"(reference=w289, error in=w262, "Path"=w281) -> (error out=w251:errorcluster, "AddFile"=w288:refnum<vi>)  [unwired: 1 in, 2 out]
            n113 = call <resource>:"CommonVIs_Wait.vi"("error in"=w251) -> ("error out"=w250:errorcluster)  [unwired: 9 in]
            n114 = call <resource>:"Error_ClearError.vi"("code"=w260, "error in (no error)"=w250) -> ("error out"=w261:errorcluster)  [unwired: 16 in, 1 out]
            n115 = invoke class="ProjectItem" method="AddFile"(reference=w278, error in=w261, "Path"=w266) -> (error out=w249:errorcluster, "AddFile"=w275:refnum<vi>)  [unwired: 1 in, 2 out]
            n116 = Unbundle By Name(w259) -> ("GetClassAttributesRef"=w257:refnum<vi>, "ClassAttributesRef"=w254:refnum<vi>)
            n117 = call <resource>:"CommonVIs_Wait.vi"("error in"=w249) -> ("error out"=w248:errorcluster)  [unwired: 9 in]
            n118 = call <resource>:"Error_ClearError.vi"("code"=w260, "error in (no error)"=w248) -> ("error out"=w252:errorcluster)  [unwired: 16 in, 1 out]
            n119 = invoke class="VI" method="Save.Instrument"(reference=w282, error in=w252) -> (reference out=w258:refnum<vi>, error out=w277:errorcluster)  [unwired: 4 in, 4 out]
            n120 = Select(t=w257, s=w251, f=w258) -> (s? t:f=w256:refnum<vi>)
            n121 = invoke class="VI" method="Save.Instrument"(reference=w270, error in=w277) -> (reference out=w255:refnum<vi>, error out=w276:errorcluster)  [unwired: 4 in, 4 out]
            n122 = Select(t=w254, s=w249, f=w255) -> (s? t:f=w253:refnum<vi>)
            n123 = Bundle By Name(cluster=w259, "GetClassAttributesRef"=w256, "ClassAttributesRef"=w253) -> (w291:T5)
            n124 = Close Reference(reference=w288, error in (no error)=w276) -> ()  [unwired: 1 out]
            n125 = Close Reference(reference=w275, error in (no error)=w276) -> ()  [unwired: 1 out]
          }
          frame "UpdateOORefInVIs" {
            n126 = property class="LVClassLibrary"(reference=w302) -> ("Path"=w300:path)  [unwired: 1 in, 2 out]
            n127 = Unbundle By Name(w304) -> ("GetClassAttributesRef"=w296:refnum<vi>)
            n128 = Build Array(w296) -> (w301:refnum<vi>[])
            n129 = Path To String(path=w300) -> (string=w299:string)
            n130 = for {
              tunnel: w301 -> [w305] mode=indexing
              shift-right: [w308] -> w297
              shift-left: w303 -> [w307]
              tunnel: w299 -> [w306]
              n131 = call <resource>:"Scripting_ReplaceOORef.vi"("ViRef"=w305, "NewLvClassFile(ProjectPath or LvClassPath)"=w306, "error in (no error)"=w307) -> ("error out"=w308:errorcluster)  [unwired: 16 in]
            }
            n132 = invoke class="VI" method="Lock State.Set"(reference=w296, error in=w297, "lockState"=T8."Not Locked" ("Lock State")) -> (reference out=w294:refnum<vi>, error out=w293:errorcluster)  [unwired: 4 in, 5 out]
            n133 = invoke class="VI" method="User Edits.Allow"(reference=w294, error in=w293) -> ()  [unwired: 1 in, 3 out]
          }
          frame "UpdateAttributes" {
            n134 = Unbundle By Name(w317) -> ("Data"=w310:T2)
            n135 = for {
              tunnel: w310 -> [w332] mode=indexing
              tunnel: [w331] -> w315 mode=indexing
              tunnel: [w330] -> w314 mode=indexing
              tunnel: [w329] -> w313 mode=indexing
              n136 = Unbundle By Name(w332) -> ("Name"=w331:string, "AttributeDataType"=w330:T1, "Array?"=w329:u16)  [unwired: 2 out]
            }
            n137 = Array Size(array=w310) -> (size(s)=w309:i32)
            n138 = case shown="1.." w309 {
              tunnel: w316 -> [_ w326]
              tunnel: w315 -> [_ w325]
              tunnel: w314 -> [_ w324]
              tunnel: w313 -> [_ w323]
              tunnel: w312 -> [w319 w321]
              tunnel: [w319 w320] -> w311
              frame 0, Default {
              }
              frame 1.. {
                n139 = call <resource>:"Scripting_PlaceControlsInClassAttribute.vi"("ClassRefnum"=w326, "ClassControl(if empty private member data will be used)"="ClassAttributes.ctl", "DeleteAllCurrentAttributesFirst(True)"=TRUE, "ControlNames"=w325, "DataTypes"=w324, "error in"=w321, "DeleteReferencesToCreatedAttributes(True)"=FALSE, "ArrayDimensions"=w323) -> ("error out"=w320:errorcluster)  [unwired: 5 in, 2 out]
              }
            }
          }
          frame "UpdateIcons" {
            w357 = u8 32 ("x")
            n140 = Unbundle By Name(w338) -> ("ClassAttributesRef"=w339:refnum<vi>, "GetClassAttributesRef"=w333:refnum<vi>)
            n141 = property class="LVClassLibrary"(reference=w340, error in=w336) -> (reference out=w345:refnum<vi>, error out=w341:errorcluster, "Member Data"=w343:refnum<vi>)
            n142 = call <resource>:"GDSLvIcon_AnalyseViIcon.vi"("ViRef/LvCLassRef/LvLibRef/ViPath"=w343, "error in (no error)"=w341) -> ("HeaderIcon"=w346:u8[][], "error out"=w342:errorcluster)  [unwired: 5 in, 11 out]
            n143 = Close Reference(reference=w343, error in (no error)=w342) -> (error out=w344:errorcluster)
            n144 = Build Array(w339, w333) -> (w334:refnum<vi>[])
            n145 = Array Size(array=w346) -> (size(s)=w352:i32[])
            n146 = call <resource>:"GDSLvClass_ReadClassColors.vi"("Library Refnum"=w345, "error in (no error)"=w344) -> ("LvClassIconSettings"=w348:T19, "error out"=w337:errorcluster)  [unwired: 12 in, 4 out]
            n147 = Unbundle By Name(w348) -> ("Frame"=w351:u32, "Body Text"=w350:u32, "Frame thickness"=w347:u8)
            n148 = Unbundle By Name(w348) -> ("ColorProtected"=w349:u32)
            n149 = Index Array(array=w352) -> (element #1=w354:i32)  [unwired: 2 in, 1 out]
            n150 = Multiply(x=w347, y=u8 2) -> (x*y=w355:u8)
            n151 = Add(x=w354, y=w355) -> (x+y=w356:i32)
            n152 = Increment(x=w356) -> (x+1=w358:i32)
            n153 = Subtract(x=w357, y=w358) -> (x-y=w359:i32)
            n154 = Subtract(x=w357, y=w355) -> (x-y=w360:u8)
            n155 = for {
              tunnel: w360 -> [_]
              tunnel: w359 -> [_]
              tunnel: w351 -> [w375]
              tunnel: w350 -> [_]
              tunnel: w349 -> [_]
              tunnel: w347 -> [w374]
              tunnel: w346 -> [w373]
              shift-right: [w366] -> w335
              shift-left: w337 -> [w365]
              tunnel: w334 -> [w362] mode=indexing
              n156 = call <resource>:"GDSLvIcon_AnalyseViIcon.vi"("ViRef/LvCLassRef/LvLibRef/ViPath"=w362, "error in (no error)"=w365) -> ("BodyIcon"=w363:u8[][], "error out"=w364:errorcluster)  [unwired: 5 in, 11 out]
              n157 = call <resource>:"GDSLvIcon_CreateIconPicture.vi"("FrameColor"=w375, "FrameThickness(1)"=w374, "HeaderIconIn"=w373, "BodyIconIn"=w363, "error in (no error)"=w364) -> ("WholeIconOut"=w368:u8[][], "error out"=w371:errorcluster)  [unwired: 9 in, 4 out]
              n158 = Reshape Array(w368, 1024 ("dimension size")) -> (w370:u8[])
              n159 = Bundle By Name(cluster=T9 {"image type"=0, "image depth"=8, "image"=[], "mask"=[], "colors"=[], "Rectangle"={"left"=0, "top"=0, "right"=32, "bottom"=32}} ("image data"), "image"=w370) -> (w372:T9)
              n160 = invoke class="VI" method="VI Icon.Set from Image Data"(reference=w362, error in=w371, "ImageData"=w372) -> (error out=w366:errorcluster)  [unwired: 3 in, 5 out]
            }
          }
          frame "CreateMethods" {
            n161 = Unbundle By Name(w379) -> ("Data"=w406:T2)
            n162 = call <resource>:"CreateWriterFromClass.vi"("ClassPath/LvClassRef"=w385, "error in"=w389) -> ("ClassWriter"=w399:refnum<class "ClassWriter.lvclass">, "LVClassRef"=w397:refnum<vi>, "error out"=w400:errorcluster)  [unwired: 15 out]
            n163 = for {
              tunnel: w406 -> [w416] mode=indexing
              shift-right: [w409] -> w405
              shift-left: string[] [] -> [w410]
              n164 = Unbundle By Name(w416) -> ("Name"=w411:string, "GetMethod"=w415:bool, "SetMethod"=w412:bool)
              n165 = case shown="True" w415 {
                tunnel: w411 -> [w423 _]
                tunnel: [w421 _] -> w414
                frame True {
                  n166 = Format Into String(format string="Get%s", w423) -> (resulting string=w422:string)  [unwired: 2 in, 1 out]
                  n167 = Build Array(w422) -> (w421:string[])
                }
                frame False {
                }
              }
              n168 = case shown="True" w412 {
                tunnel: w411 -> [w419 _]
                tunnel: [w417 _] -> w413
                frame True {
                  n169 = Format Into String(format string="Set%s", w419) -> (resulting string=w418:string)  [unwired: 2 in, 1 out]
                  n170 = Build Array(w418) -> (w417:string[])
                }
                frame False {
                }
              }
              n171 = Build Array (concatenate)(w410, w414, w413) -> (w409:string[])
            }
            n172 = call <resource>:"GDSLvClass_ReadClassType.vi"("Class Refnum In"=w397, "error in (no error)"=w400) -> ("ClassSettings"=w394:T14)  [unwired: 17 out]
            n173 = Unbundle By Name(w394) -> ("ClassTemplateUsed"=w395:string)
            n174 = Empty String/Path?(string/path=w395) -> (empty?=w392:bool)
            n175 = To More Specific Class(target class=refnum<class "ClassWriterNative.lvclass"> refnum ("reference in"), reference=w399, error in=w400) -> (specific class reference=w402:refnum<class "ClassWriterNative.lvclass">)  [unwired: 1 out]
            n176 = Select(t="BaseTemplate", s=w392, f=w395) -> (s? t:f=w396:string)
            n177 = call-dynamic "GetTemplatePath.vi"("reference in"=w402, "ClassTemplateSubDirectory"=w396, "error in (no error)"=w400) -> ("reference out"=w390:refnum<class "ClassWriterNative.lvclass">, "MethodTemplatePathOut"=w398:path, "error out"=w403:errorcluster)  [unwired: 14 out]
            n178 = call <resource>:"GetClassTemplateMethods.vi"("MethodTemplatePath"=w398, "error in"=w403) -> ("PropertyMethodPaths"=w388:path[], "error out"=w391:errorcluster)  [unwired: 1 in, 15 out]
            n179 = for {
              tunnel: w385 -> [w445]
              shift-right: [w447] -> w408
              shift-left: w391 -> [w444]
              shift-right: [w446] -> w407
              shift-left: w390 -> [w443]
              tunnel: w405 -> [w434] mode=indexing
              tunnel: w388 -> [w438]
              n180 = Match Pattern(string=w434, regular expression="^[Ss][Ee][Tt]") -> (offset past match=w436:i32)  [unwired: 1 in, 3 out]
              n181 = String Subset(string=w434, offset (0)=3) -> (substring=w426:string)  [unwired: 1 in]
              n182 = Greater Or Equal To 0?(x=w436) -> (x >= 0?=w432:bool)
              n183 = Boolean To (0,1)(Boolean=w432) -> (0, 1=w435:i16)
              n184 = Index Array(array=w438, index=w435) -> (element=w440:path)
              n185 = Strip Path(path=w440) -> (name=w439:string)  [unwired: 1 out]
              n186 = Select(t="This method reads the class attribute %s" ("format string"), s=w432, f="This method writes the class attribute %s" ("format string")) -> (s? t:f=w429:string)
              n187 = Format Into String(format string=w429, w426) -> (resulting string=w428:string)  [unwired: 2 in, 1 out]
              n188 = Concatenate Strings("ClassAttribute§" ("format string"), w426) -> (w425:string)
              n189 = Bundle By Name(cluster=T10 {"MethodName"="", "RelativeMethodPath"=path "", "MethodDescription"="", "Scope/Visibility"=enum."Public", "MethodTemplateName"="", "IconOut"=[], "RelativeProjectClassPath"="", "OpenViAfterCreation"=FALSE, "DynamicDispatchVi"=FALSE, "ExtraCreateParameters"=variant, "MustOverride"=FALSE, "MustCallParent"=FALSE, "IconDetails"={"IconSize"=enum."Full", "ImageRows(32)"=0, "ConnectorPaneHeight"=[]}, "AF-Option"=variant, "TemplatePath"=path ""} ("CreateMethodData"), "ExtraCreateParameters"=w425, "MethodName"=w434, "MethodDescription"=w428, "MethodTemplateName"=w439) -> (w441:T10)
              n190 = call-dynamic "CreateMethod.vi"("ClassWriterNative.lvclass"=w443, "ClassItemRefIn"=w445, "CreateMethodData"=w441, "error in (no error)"=w444) -> ("ClassWriterNative.lvclass 2"=w446:refnum<class "ClassWriterNative.lvclass">, "error out"=w447:errorcluster)  [unwired: 13 in, 1 out]
            }
            n191 = call-dynamic "Destroy.vi"("ClassWriterNative"=w407, "error in (no error)"=w408) -> ("error out"=w387:errorcluster)  [unwired: 17 in]
            n192 = call <resource>:"GDSLvClass_GetClassMethod.vi"("Class Refnum In"=w385, "VINames"=string[] ["_GetObjectStatus.vi"], "error in (no error)"=w387) -> ("ViPaths"=w380:path[], "error out"=w386:errorcluster)  [unwired: 13 in, 2 out]
            n193 = Index Array(array=w380) -> (element=w377:path)  [unwired: 1 in]
            n194 = Bundle By Name(cluster=w379, "GetObjectStatus"=w377) -> (w378:T5)
            n195 = Empty String/Path?(string/path=w377) -> (empty?=w376:bool)
            n196 = Select(t="CloseRefs", s=w376, f="UpdateGetObjectStatus") -> (s? t:f=w381:string)
          }
          frame "UpdateGetObjectStatus" {
            n197 = Unbundle By Name(w460) -> ("Application"=w459:refnum<vi>)
            n198 = Unbundle By Name(w460) -> ("GetObjectStatus"=w457:path, "ProtectedFolder"=w493:path)
            n199 = call <resource>:"GDSLvClass_GetClassMethod.vi"("Class Refnum In"=w475, "VINames"=string[] ["_GetClassAttributes.vi"] ("VIsToSerachFor/ViName"), "error in (no error)"=w476) -> ("ViPaths"=w477:path[], "error out"=w458:errorcluster)  [unwired: 13 in, 2 out]
            n200 = Index Array(array=w477) -> (element #1=w480:path, element #2=w479:path)  [unwired: 2 in]
            n201 = call <resource>:"Scripting_OpenViRef.vi"("error in"=w458, "ViPath/ViName"=w457, "AppRef"=w459) -> ("error out"=w455:errorcluster, "vi reference"=w454:refnum<vi>)  [unwired: 7 in]
            n202 = Empty String/Path?(string/path=w480) -> (empty?=w478:bool)
            n203 = invoke class="VI" method="Lock State.Set"(reference=w454, error in=w455, "lockState"=T8."Not Locked" ("Lock State")) -> (reference out=w453:refnum<vi>, error out=w452:errorcluster)  [unwired: 4 in, 5 out]
            n204 = Select(t=w479, s=w478, f=w480) -> (s? t:f=w468:path)
            n205 = call <resource>:"Scripting_FindObjectsOnDiagram.vi"("ViRef(Ignored If Not Wired)"=w453, "NodeTypesToSearchFor"=string[] ["ClusterConstant"], "Don'tSearchSubStructures(False)"=TRUE, "error in (no error)"=w452) -> ("Nodes"=w450:refnum<vi>[], "error out"=w484:errorcluster)  [unwired: 14 in]
            n206 = for {
              tunnel: w450 -> [w527] mode=indexing
              shift-right: [w523] -> w451
              shift-left: w484 -> [w524]
              tunnel: [w522] -> w490 mode=indexing
              n207 = To More Specific Class(target class=refnum<vi> refnum ("WhileLoop"), reference=w527, error in=w524) -> (specific class reference=w526:refnum<vi>, error out=w525:errorcluster)
              n208 = property class="ClustCnst"(reference=w526, error in=w525) -> (error out=w523:errorcluster, "Label.Text"=w522:string)  [unwired: 1 out]
            }
            n209 = Empty String/Path?(string/path=w468) -> (empty?=w469:bool)
            n210 = Build Path(base path=w493, name or relative path="ClassAttributes.ctl") -> (appended path=w487:path)
            n211 = Search 1D Array(1D array=w490, element="ClassAttributes") -> (index of element=w491:i32)  [unwired: 1 in]
            n212 = Delete From Array(array=w450, index=w491) -> (deleted portion=w492:refnum<vi>, array with subset deleted=w449:refnum<vi>[])  [unwired: 1 in]
            n213 = invoke class="GObj" method="Replace"(reference=w492, error in=w451, "Path"=w487) -> (error out=w489:errorcluster, "Replace"=w488:refnum<vi>)  [unwired: 3 in, 4 out]
            n214 = Close Reference(reference=w488, error in (no error)=w489) -> (error out=w494:errorcluster)
            n215 = Close Reference(reference=w449, error in (no error)=w494) -> (error out=w470:errorcluster)
            n216 = call <resource>:"Scripting_FindVisOnDiagram.vi"("ViRef"=w453, "VIsToSerachFor/ViName"=string[] ["_GetAttributes.vi$"], "error in (no error)"=w470) -> ("VisFound"=w472:refnum<vi>[], "error out"=w471:errorcluster)  [unwired: 15 in]
            n217 = for {
              tunnel: [w515] -> w473 mode=indexing
              shift-right: [w514] -> w448
              shift-left: w471 -> [w513]
              tunnel: w472 -> [w512] mode=indexing
              tunnel: w469 -> [w506]
              tunnel: w468 -> [w505]
              w510 = refnum<vi> refnum  # Node
              n218 = To More Specific Class(target class=w510, reference=w512) -> (specific class reference=w511:refnum<vi>)  [unwired: 1 in, 1 out]
              n219 = property class="Node"(reference=w511, error in=w513) -> ("Desc"=w509:string)  [unwired: 2 out]
              n220 = Equal?(x=w509, y="ClassAttribute") -> (x = y?=w507:bool)
              n221 = Compound Arithmetic op=AND(w507, invert w506) -> (w504:bool)
              n222 = case shown="True" w504 {
                tunnel: [_ w521] -> w515
                tunnel: [w516 w520] -> w514
                tunnel: w513 -> [w516 w519]
                tunnel: w512 -> [_ w518]
                tunnel: w505 -> [_ w517]
                frame False {
                }
                frame True {
                  n223 = invoke class="GObj" method="Replace"(reference=w518, error in=w519, "Path"=w517) -> (error out=w520:errorcluster, "Replace"=w521:refnum<vi>)  [unwired: 3 in, 4 out]
                }
              }
            }
            n224 = Close Reference(reference=w472, error in (no error)=w448) -> ()  [unwired: 1 out]
            n225 = Close Reference(reference=w473, error in (no error)=w448) -> ()  [unwired: 1 out]
            n226 = invoke class="VI" method="BD.Remove Bad Wires"(reference=w453, error in=w448) -> (reference out=w462:refnum<vi>, error out=w463:errorcluster)  [unwired: 1 in, 1 out]
            n227 = call <resource>:"Scripting_FindNodeOnDiagram.vi"("ViRef(Ignored If Not Wired)"=w462, "NodeTypesToSearchFor"=string[] ["DisableStructure"], "error in (no error)"=w463) -> ("Nodes"=w467:refnum<vi>[], "error out"=w465:errorcluster)  [unwired: 15 in]
            n228 = for {
              tunnel: w467 -> [w503] mode=indexing
              shift-right: [w496] -> w466
              shift-left: w465 -> [w499]
              w501 = i16 0 ("number")
              w502 = refnum<vi> refnum  # DisableStructure
              n229 = To More Specific Class(target class=w502, reference=w503, error in=w499) -> (specific class reference=w497:refnum<vi>, error out=w498:errorcluster)
              n230 = To Word Integer(number=w501) -> (16bit integer=w500:i16)
              n231 = property class="DisableStructure"(reference=w497, error in=w498, "VisFrame"=w501, "ActiveFrame"=w500) -> (error out=w496:errorcluster)  [unwired: 1 out]
            }
            n232 = Close Reference(reference=w467, error in (no error)=w466) -> (error out=w461:errorcluster)
          }
        }
        n233 = Equal?(x=w125, y="Exit") -> (x = y?=w128:bool)
        n234 = Select(t="Error", s=w124, f=w125) -> (s? t:f=w129:string)
      }
    }
    frame "CreatePatternMethod" {
      w529 = "Init"
      n235 = property class="VI"(error in=w531, "Front Panel.Open"=FALSE ("Front Panel Window:Open")) -> (error out=w530:errorcluster)  [unwired: 1 in, 1 out]
      n236 = while {
        shift-right: [w545] -> w537
        shift-left: w530 -> [w552]
        shift-right: [w550] -> _
        shift-left: w529 -> [w551]
        shift-right: [w544] -> _
        shift-left: _ -> [w543]
        tunnel: w536 -> [w542]
        tunnel: w535 -> [w541]
        tunnel: w534 -> [w540]
        tunnel: w533 -> [w539]
        shift-left: w529 -> [w538]
        stop <- w549 stop-if-true
        n237 = case shown="\"Find_GetInstanceVI\"" w551 {
          tunnel: w552 -> [w581 w589 w616]
          tunnel: [w573 w587 w617] -> w545
          tunnel: [w571 "ReplaceGetClassAttributes" "Exit"] -> w546
          tunnel: [w584 w592 w619] -> w544
          tunnel: w543 -> [_ w592 w619]
          tunnel: w542 -> [w583 _ _]
          tunnel: w541 -> [_ _ _]
          tunnel: w540 -> [w582 _ _]
          tunnel: w539 -> [w574 w590 w618]
          tunnel: w538 -> [_ _ _]
          frame "Init" {
            n238 = Variant To Data(error in=w581, type=cluster{path, "VI":refnum<vi>, "Name":string} {path "", "VI"=refnum, "Name"=""} ("cluster"), Variant=w583) -> (data=w562:cluster{path, "VI":refnum<vi>, "Name":string}, error out=w563:errorcluster)
            n239 = Unbundle(w562) -> (w560:path, "VI"=w561:refnum<vi>)  [unwired: 1 out]
            n240 = call <resource>:"GDSLvClass_ReadClassType.vi"("Class Refnum In"=w574, "error in (no error)"=w563) -> ("ClassSettings"=w580:T14, "error out"=w573:errorcluster)  [unwired: 15 in, 1 out]
            n241 = Unbundle By Name(w580) -> ("ConnectorPanePattern"=w579:string, "ClassTemplateUsed"=w578:string)
            n242 = To Lower Case(string=w578) -> (all lower case string=w576:string)
            n243 = case shown="\"0\", Default" w579 {
              tunnel: ["4x4x4" "6x8x6"] -> w558
              frame "0", Default {
              }
              frame "1", "2" {
              }
            }
            n244 = Match Pattern(string=w576, regular expression="singleton" ("search string")) -> (offset past match=w577:i32)  [unwired: 1 in, 3 out]
            n245 = Greater Or Equal To 0?(x=w577) -> (x >= 0?=w572:bool)
            n246 = Current VI's Path() -> (path=w569:path)
            n247 = Strip Path(path=w569) -> (stripped path=w568:path)  [unwired: 1 out]
            n248 = Format Into String(format string="ClassAttributes_ReadClassAttributes_%s.vi" ("name or relative path"), w558) -> (resulting string=w565:string)  [unwired: 2 in, 1 out]
            n249 = Build Path(base path=w568, name or relative path="ClassAttributes_SubVIs") -> (appended path=w556:path)
            n250 = Format Into String(format string="ClassAttributes_GetClassAttributes_%s.vi" ("name or relative path"), w558) -> (resulting string=w559:string)  [unwired: 2 in, 1 out]
            n251 = Build Path(base path=w556, name or relative path=w565) -> (appended path=w564:path)
            n252 = Build Path(base path=w556, name or relative path=w559) -> (appended path=w555:path)
            n253 = Select(t="Find_GetInstanceVI", s=w572, f="ReplaceGetClassAttributes") -> (s? t:f=w571:string)
            n254 = Bundle By Name(cluster=w582, "MethodTemplate"=w560, "VI"=w561, "SupportFolder"=w556, "VI_ToFind"=w564, "GetClassAttributes.vi"=w555) -> (w584:T5)
          }
          frame "Find_GetInstanceVI" {
            n255 = Unbundle By Name(w592) -> ("VI_ToFind"=w595:path, "VI"=w588:refnum<vi>)
            n256 = Build Array(w595) -> (w594:path[])
            n257 = call <resource>:"GDSLvClass_GetClassMethod.vi"("Class Refnum In"=w590, "VINames"=string[] ["_GetInstance.vi$"] ("VIsToSerachFor/ViName"), "error in (no error)"=w589) -> ("ViPaths"=w601:path[], "error out"=w596:errorcluster)  [unwired: 13 in, 2 out]
            n258 = call <resource>:"Scripting_FindVisOnDiagram.vi"("ViRef"=w588, "VIsToSerachFor/ViName"=w594, "error in (no error)"=w596) -> ("VisFound"=w598:refnum<vi>[], "error out"=w597:errorcluster)  [unwired: 15 in]
            n259 = Index Array(array=w601) -> (element=w593:path)  [unwired: 1 in]
            n260 = Index Array(array=w598) -> (element=w599:refnum<vi>)  [unwired: 1 in]
            n261 = invoke class="GObj" method="Replace"(reference=w599, error in=w597, "Path"=w593) -> (error out=w591:errorcluster, "Replace"=w600:refnum<vi>)  [unwired: 3 in, 4 out]
            n262 = Close Reference(reference=w598, error in (no error)=w591) -> ()  [unwired: 1 out]
            n263 = Close Reference(reference=w600, error in (no error)=w591) -> (error out=w587:errorcluster)
          }
          frame "ReplaceGetClassAttributes", Default {
            n264 = Unbundle By Name(w619) -> ("GetClassAttributes.vi"=w609:path, "VI"=w604:refnum<vi>)
            n265 = Build Array(w609) -> (w608:path[])
            n266 = call <resource>:"GDSLvClass_GetClassMethod.vi"("Class Refnum In"=w618, "VINames"=string[] ["GetClassAttributes.vi$"] ("VIsToSerachFor/ViName"), "error in (no error)"=w616) -> ("ViPaths"=w606:path[], "error out"=w607:errorcluster)  [unwired: 13 in, 2 out]
            n267 = Index Array(array=w606) -> (element=w605:path)  [unwired: 1 in]
            n268 = call <resource>:"Scripting_FindVisOnDiagram.vi"("ViRef"=w604, "VIsToSerachFor/ViName"=w608, "error in (no error)"=w607) -> ("VisFound"=w612:refnum<vi>[], "error out"=w611:errorcluster)  [unwired: 15 in]
            n269 = Index Array(array=w612) -> (element=w614:refnum<vi>)  [unwired: 1 in]
            n270 = invoke class="GObj" method="Replace"(reference=w614, error in=w611, "Path"=w605) -> (error out=w615:errorcluster, "Replace"=w613:refnum<vi>)  [unwired: 3 in, 4 out]
            n271 = Close Reference(reference=w612, error in (no error)=w615) -> ()  [unwired: 1 out]
            n272 = Close Reference(reference=w613, error in (no error)=w615) -> (error out=w610:errorcluster)
            n273 = invoke class="VI" method="Save.Instrument"(reference=w604, error in=w610) -> (error out=w617:errorcluster)  [unwired: 4 in, 5 out]
          }
        }
        n274 = Equal?(x=w546, y="Exit") -> (x = y?=w549:bool)
        n275 = Select(t="Error", s=w545, f=w546) -> (s? t:f=w550:string)
      }
    }
    frame "UpdatePattern" {
    }
    frame "RemovePattern" {
    }
  }
  "error out" <- w8
  "DataOut" <- w5
  "Cancelled" <- w6
  "Name" <- "Class Attributes" ("Name")
